vi "命令格式.vi"(11 "站号":u16(ring)=1 items=["null"=0, "总磷"=1, "总氮"=2, "氨氮"=3, "CODMn"=21, "CODCr"=22]) -> (3 "命令格式":u16)   [LabVIEW 2016, in "质控单元V4.lvlib"]
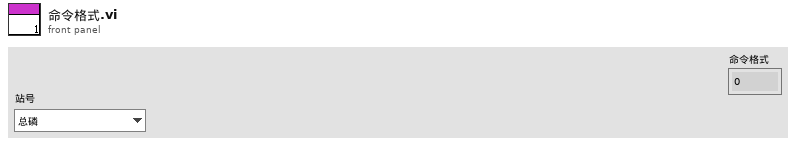
[diagram p1: front panel]
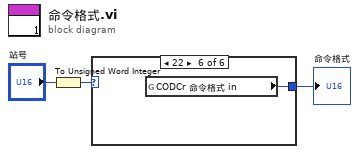
[diagram p0: block diagram]
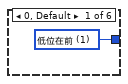
[diagram p2: hidden frame]
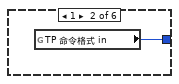
[diagram p3: hidden frame]
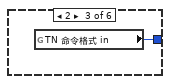
[diagram p4: hidden frame]
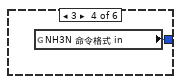
[diagram p5: hidden frame]
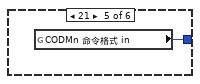
[diagram p6: hidden frame]
diagram:
  n1 = To Unsigned Word Integer(number="站号") -> (unsigned 16bit integer=w3:u16)
  n2 = case shown="22" w3 {
    tunnel: [w4 w5 w6 w7 w8 w9] -> w2
    frame 0, Default {
      w4 = u16 1 items=["自动", "低位在前", "低位在后"] ("CODCr 命令格式 in")
    }
    frame 1 {
      n3 = global read "系统交互.vi" "TP 命令格式 in"() -> (w5:u16)
    }
    frame 2 {
      n4 = global read "系统交互.vi" "TN 命令格式 in"() -> (w6:u16)
    }
    frame 3 {
      n5 = global read "系统交互.vi" "NH3N 命令格式 in"() -> (w7:u16)
    }
    frame 21 {
      n6 = global read "系统交互.vi" "CODMn 命令格式 in"() -> (w8:u16)
    }
    frame 22 {
      n7 = global read "系统交互.vi" "CODCr 命令格式 in"() -> (w9:u16)
    }
  }
  "命令格式" <- w2
